vi "Read Frequency Limits.vi"(0 "VISA resource name":refnum<visa-resource-name>, 11 "error in (no error)":errorcluster) -> (4 "VISA resource name out":refnum<visa-resource-name>, 6 "Frequency Low Limit (Hz)":dbl, 8 "Frequency High Limit (Hz)":dbl, 15 "error out":errorcluster)   [LabVIEW 2014, in "eec 6700.lvlib"]
doc: "Reads the Frequency limits set in the power source instrument.\n\nNote : Check whether the instrument is in Program or Manual mode."
uses:
  <instrlib>/eec 6700/eec 6700.lvlib
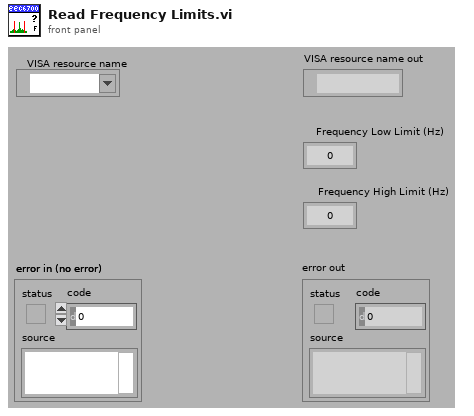
[diagram p1: front panel]
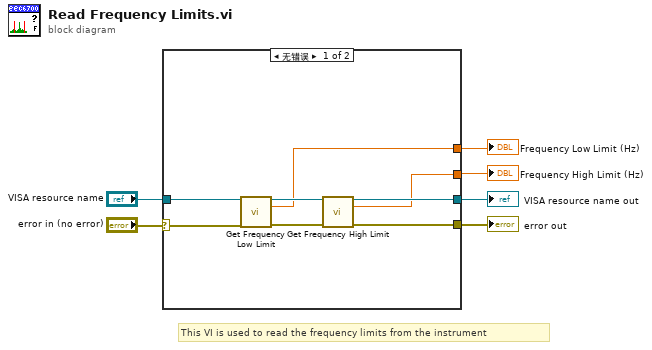
[diagram p0: block diagram]
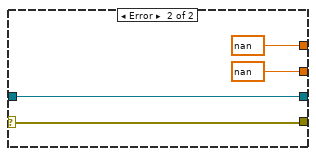
[diagram p2: hidden frame]
diagram:
  # "This VI is used to read the frequency limits from the instrument"
  n1 = case shown="无错误" "error in (no error)" {
    selector: "error in (no error)" -> [w14 w15]
    tunnel: [w12 w15] -> w5
    tunnel: [w11 w16] -> w4
    tunnel: "VISA resource name" -> [w9 w16]
    tunnel: [w7 nan ("Voltage Low Limit")] -> w2
    tunnel: [w8 nan ("Voltage Low Limit")] -> w1
    frame No Error {
      n2 = call <instrlib>:"Get Frequency Low Limit.vi"("VISA resource name"=w9, "error in (no error)"=w14) -> ("VISA resource name out"=w10:refnum<visa-resource-name>, "Frequency Low Limit (Hz)"=w7:dbl, "error out"=w13:errorcluster)  [unwired: 11 in]
      n3 = call <instrlib>:"Get Frequency High Limit.vi"("VISA resource name"=w10, "error in (no error)"=w13) -> ("VISA resource name out"=w11:refnum<visa-resource-name>, "Frequency High Limit (Hz)"=w8:dbl, "error out"=w12:errorcluster)  [unwired: 11 in]
    }
    frame Error {
    }
  }
  "error out" <- w5
  "VISA resource name out" <- w4
  "Frequency High Limit (Hz)" <- w1
  "Frequency Low Limit (Hz)" <- w2
